vi "addDelayMilliseconds.vi"(8 "error in (no error)":errorcluster, 10 "Milliseconds":u16, 11 "Modbus in":refnum<class "Modbus.lvclass">) -> (0 "error out":errorcluster, 3 "Modbus out":refnum<class "Modbus.lvclass">)   [LabVIEW 2016, in "RTModbus.lvlib" / "Modbus.lvclass"]
uses:
  Modbus.lvclass
  DataTypes/TxFrame.ctl
  RTModbus.lvlib
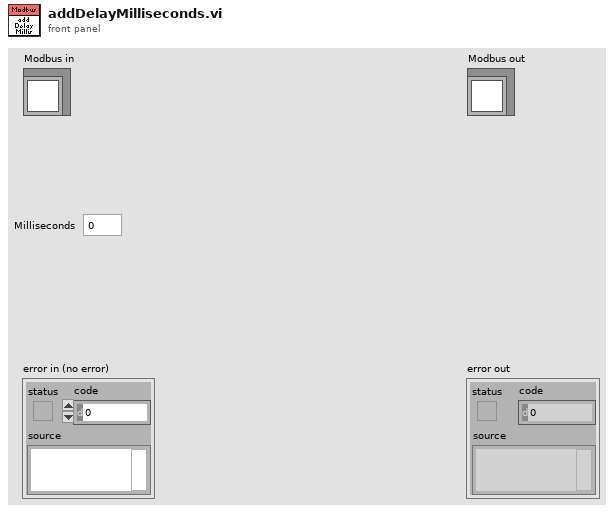
[diagram p1: front panel]
types:
  T1 = typedef "RTModbus.lvlib/TxFrame.ctl" = cluster{"Data":u8[], "WaitForTrigger":bool, "WaitForRx":u16, "TriggerIRQ":bool, "DelayMicroseconds":u16, "DelayMilliseconds":u16, "Timestamp":bool}
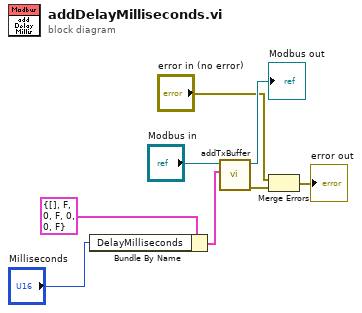
[diagram p0: block diagram]
diagram:
  n1 = Bundle By Name(cluster=T1 {"Data"=[], "WaitForTrigger"=FALSE, "WaitForRx"=0, "TriggerIRQ"=FALSE, "DelayMicroseconds"=0, "DelayMilliseconds"=0, "Timestamp"=FALSE} ("Frame"), "DelayMilliseconds"="Milliseconds") -> (w7:T1)
  n2 = call-dynamic "addTxBuffer.vi"("TxFrame"=w7, "Modbus in"="Modbus in") -> ("error out"=w3:errorcluster, "Modbus out"=→"Modbus out":refnum<class "Modbus.lvclass">)  [unwired: 8 in]
  n3 = Merge Errors("error in (no error)", w3) -> (→"error out":errorcluster)
